vi "Read singleplayer.vi"(8 "error in (no error)":errorcluster, 11 "Pong in":refnum<class "Pong.lvclass">) -> (0 "error out":errorcluster, 2 "singleplayer":bool, 3 "Pong out":refnum<class "Pong.lvclass">)   [LabVIEW 2019, in "RT_Game.lvlib" / "Pong.lvclass"]
uses:
  Pong.lvclass
  Pong.lvclass/Pong.ctl
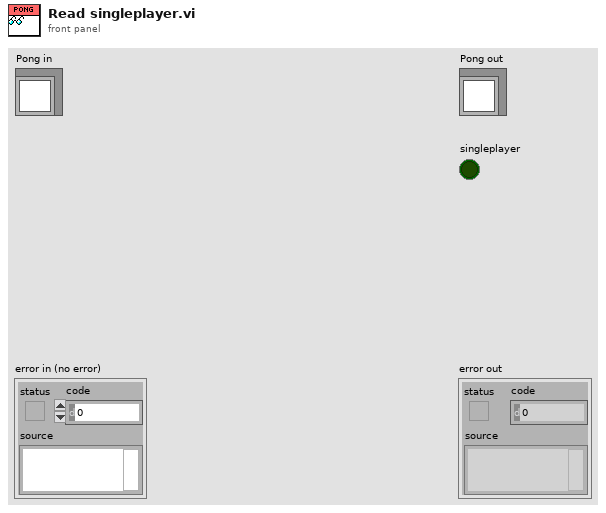
[diagram p1: front panel]
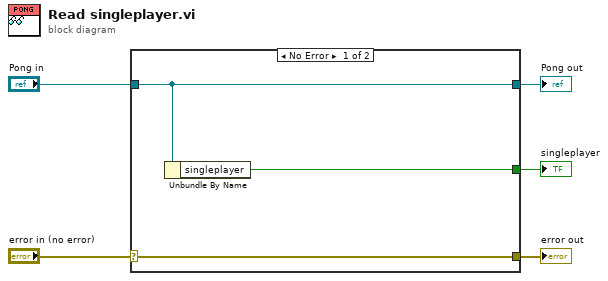
[diagram p0: block diagram]
diagram:
  n1 = case shown="No Error" "error in (no error)" {
    selector: "error in (no error)" -> [w8 w9]
    tunnel: [w8 w9] -> w4
    tunnel: [w7 w10] -> w2
    tunnel: "Pong in" -> [w7 w10]
    tunnel: [w6 _] -> w1
    frame No Error {
      n2 = Unbundle By Name(w7) -> ("singleplayer"=w6:bool)
    }
    frame Error {
    }
  }
  "error out" <- w4
  "Pong out" <- w2
  "singleplayer" <- w1
